vi "open_swerve.vi"(8 "error in (no error)":errorcluster) -> (0 "error out":errorcluster)   [LabVIEW 2020]
uses:
  Status Frame Stuff/Pigeon Status Config Array.ctl
  <vilib>/Rock Robotics/WPI/ThirdParty/Phoenix-LabVIEW/Pigeon IMU/CTRE_PigeonIMU_StatusFrameRate.ctl
  Status Frame Stuff/STATUS_Period.ctl
  <vilib>/Rock Robotics/WPI/ThirdParty/Phoenix-LabVIEW/Pigeon IMU/CTRE_PigeonIMU_Open_CAN.vi
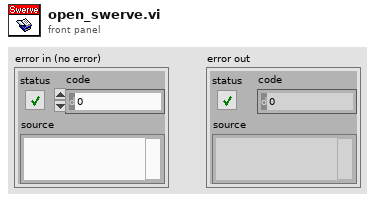
[diagram p1: front panel]
types:
  T1 = typedef "Pigeon Status Config Array.ctl" = cluster{"Status Frame Enum":T2, "STATUS_Period":T3}[]
  T2 = typedef "CTRE_PigeonIMU_StatusFrameRate.ctl" = u32
  T3 = typedef "STATUS_Period.ctl" = i32
  T4 = typedef "CTRE_PigeonIMU_DeviceRef.ctl" = cluster{"DeviceStatus":errorcluster, "Device Number":u8, "Type":T5, "Device ID":u32, "Handle":u64, "UsageFrame":u32, "Library Path":path}
  T5 = typedef "CTRE_PigeonIMU_ConnectionType.ctl" = u32
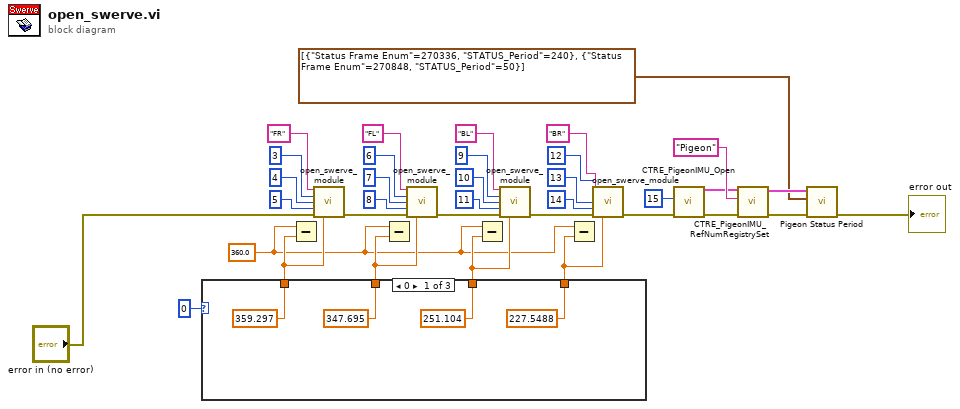
[diagram p0: block diagram]
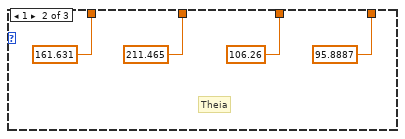
[diagram p2: hidden frame]
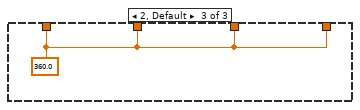
[diagram p3: hidden frame]
diagram:
  w27 = 360.0 ("Encoder Offset (Deg)")
  n1 = case shown="0" u8 0 ("Drive CAN ID") {
    tunnel: [359.297 ("Encoder Offset (Deg)") 161.631 ("Encoder Offset (Deg)") w44] -> w29
    tunnel: [347.695 ("Encoder Offset (Deg)") 211.465 ("Encoder Offset (Deg)") w44] -> w30
    tunnel: [251.104 ("Encoder Offset (Deg)") 106.26 ("Encoder Offset (Deg)") w44] -> w31
    tunnel: [227.5488 ("Encoder Offset (Deg)") 95.8887 ("Encoder Offset (Deg)") w44] -> w32
    frame 0 {
    }
    frame 1 {
      # "Theia"
    }
    frame 2, Default {
      w44 = 360.0 ("Encoder Offset (Deg)")
    }
  }
  n2 = Subtract(x=w27, y=w29) -> ()  [unwired: 1 out]
  n3 = call "open_swerve_module.vi"("Module Suffix"="FR", "Drive CAN ID"=u8 3, "Azimuth CAN ID"=u8 4 ("Drive CAN ID"), "Encoder CAN ID"=u8 5 ("Drive CAN ID"), "error in"="error in (no error)", "Encoder Offset (Deg)"=w29) -> ("error out"=w15:errorcluster)  [unwired: 9 in]
  n4 = Subtract(x=w27, y=w30) -> ()  [unwired: 1 out]
  n5 = call "open_swerve_module.vi"("Module Suffix"="FL", "Drive CAN ID"=u8 6, "Azimuth CAN ID"=u8 7 ("Drive CAN ID"), "Encoder CAN ID"=u8 8 ("Drive CAN ID"), "error in"=w15, "Encoder Offset (Deg)"=w30) -> ("error out"=w20:errorcluster)  [unwired: 9 in]
  n6 = Subtract(x=w27, y=w31) -> ()  [unwired: 1 out]
  n7 = call "open_swerve_module.vi"("Module Suffix"="BL", "Drive CAN ID"=u8 9, "Azimuth CAN ID"=u8 10 ("Drive CAN ID"), "Encoder CAN ID"=u8 11 ("Drive CAN ID"), "error in"=w20, "Encoder Offset (Deg)"=w31) -> ("error out"=w25:errorcluster)  [unwired: 9 in]
  n8 = Subtract(x=w27, y=w32) -> ()  [unwired: 1 out]
  n9 = call "open_swerve_module.vi"("Module Suffix"="BR", "Drive CAN ID"=u8 12, "Azimuth CAN ID"=u8 13 ("Drive CAN ID"), "Encoder CAN ID"=u8 14 ("Drive CAN ID"), "error in"=w25, "Encoder Offset (Deg)"=w32) -> ("error out"=w26:errorcluster)  [unwired: 9 in]
  n10 = call-poly <vilib>:"CTRE_PigeonIMU_Open.vi"("error in"=w26, "Device Number"=u8 15) -> ("error out"=w5:errorcluster, "PigeonIMUDevRef"=w6:T4)  [unwired: 8 in]
  n11 = call <vilib>:"CTRE_PigeonIMU_RefNumRegistrySet.vi"("error in (no error)"=w5, "refnum name"="Pigeon", "PigeonIMUDevRef"=w6) -> ("error out"=w35:errorcluster, "PigeonIMUDevRef"=w34:T4)  [unwired: 7 in]
  n12 = call "Pigeon Status Period.vi"("error in (no error)"=w35, "Pigeon Status Config Array"=T1 [{"Status Frame Enum"=270336, "STATUS_Period"=240}, {"Status Frame Enum"=270848, "STATUS_Period"=50}], "PigeonIMUDevRef"=w34) -> ("error out"=→"error out":errorcluster)  [unwired: 7 in, 1 out]
